vi "Test wait 2.vi"(8 "error in (no error)":errorcluster, 11 "Test Case In":refnum<class "Waiting Test 3.lvclass">) -> (0 "error out":errorcluster, 3 "Test Case Out":refnum<class "Waiting Test 3.lvclass">)   [LabVIEW 2020, in "Waiting Test 3.lvclass"]
uses:
  Waiting Test 3.lvclass
  Waiting Test 3.lvclass/Waiting Test 3.ctl
  <vilib>/Astemes/LUnit/Test Case.lvclass
  C:/Program Files (x86)/National Instruments/LabVIEW 2020/vi.lib/Astemes/LUnit/Test Case.lvclass
  C:/Users/anton/Documents/GitHub/LUnit/sandbox/Benchmark/LUnit Delaying/Waiting Test 3/Waiting Test 3.lvclass
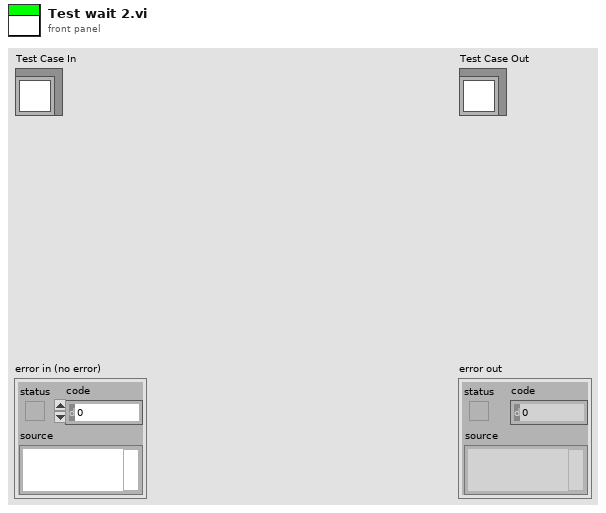
[diagram p1: front panel]
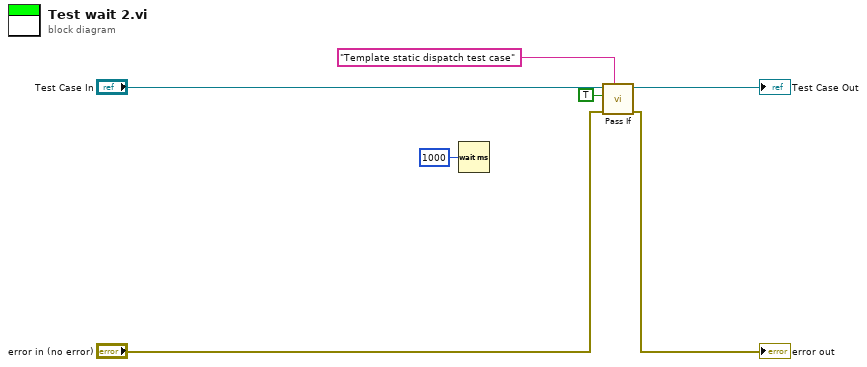
[diagram p0: block diagram]
diagram:
  n1 = Wait (ms)(milliseconds to wait=u32 1000) -> ()  [unwired: 1 out]
  n2 = call <vilib>:"Pass If.vi"("Description"="Template static dispatch test case", "error in (no error)"="error in (no error)", "Pass?"=TRUE, "LUnit Test Case In"="Test Case In") -> ("error out"=→"error out":errorcluster, "LUnit Test Case Out"=→"Test Case Out":refnum<class "Waiting Test 3.lvclass">)  [unwired: 6 in]
